vi "S_c.vi"(1 "w_in":dbl) -> (0 "w_out":dbl)   [LabVIEW 2019]
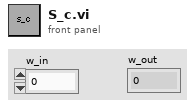
[diagram p1: front panel]
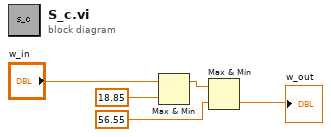
[diagram p0: block diagram]
diagram:
  n1 = Max & Min(x="w_in", y=18.85) -> (max(x,y)=w3:dbl)  [unwired: 1 out]
  n2 = Max & Min(x=w3, y=56.55) -> (min(x,y)=→"w_out":dbl)  [unwired: 1 out]
